vi "Mass Compile Helper.vi"() -> ()   [LabVIEW 2011, in "LVH-Toolbox.lvlib" / "LVH-SystemTools.lvlib"]
uses:
  LVH-SystemTools.lvlib
panel:
  in  "Error In":errorcluster
  out "Error Out":errorcluster
  # "Mass Compiling...."
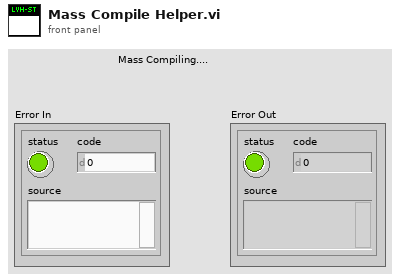
[diagram p1: front panel]
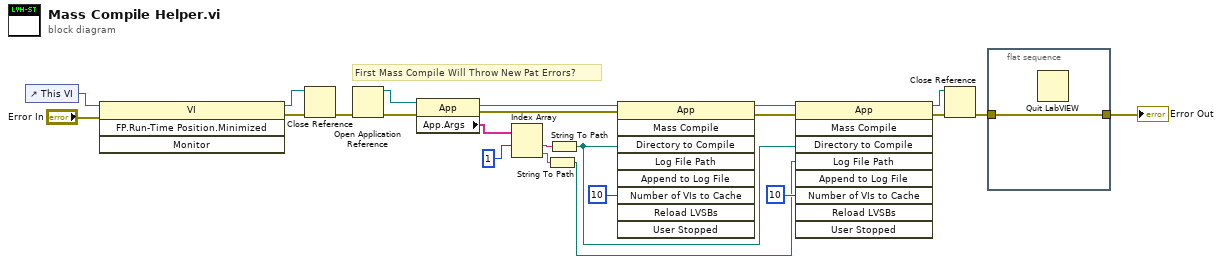
[diagram p0: block diagram]
diagram:
  # "First Mass Compile Will Throw New Pat Errors?"
  n1 = control-ref of="This VI"() -> (w5:refnum<vi>)
  n2 = invoke class="VI" method="FP.Run-Time Position.Minimized"(reference=w5, error in="Error In") -> (reference out=w2:refnum<vi>, error out=w3:errorcluster)  [unwired: 2 in, 2 out]
  n3 = Close Reference(reference=w2, error in (no error)=w3) -> (error out=w1:errorcluster)
  n4 = Open Application Reference(8:w1) -> (0:w13:errorcluster, 3:w15:refnum<vi>)  [unwired: 3 in]
  n5 = property class="App"(reference=w15, error in=w13) -> (reference out=w14:refnum<vi>, error out=w12:errorcluster, "App.Args"=w11:string[])
  n6 = Index Array(array=w11, index #1=1 ("index")) -> (element #1=w7:string, element #2=w6:string)  [unwired: 1 in]
  n7 = String To Path(string=w6) -> (path=w8:path)
  n8 = String To Path(string=w7) -> (path=w9:path)
  n9 = invoke class="App" method="Mass Compile"(reference=w14, error in=w12, "Directory to Compile"=w9, "Number of VIs to Cache"=u32 10) -> (reference out=w22:refnum<vi>, error out=w23:errorcluster)  [unwired: 5 in, 7 out]
  n10 = invoke class="App" method="Mass Compile"(reference=w22, error in=w23, "Directory to Compile"=w9, "Log File Path"=w8, "Number of VIs to Cache"=u32 10) -> (reference out=w20:refnum<vi>, error out=w21:errorcluster)  [unwired: 4 in, 7 out]
  n11 = Close Reference(reference=w20, error in (no error)=w21) -> (error out=w16:errorcluster)
  n12 = flat-sequence {
    tunnel: [w24] -> w17
    tunnel: w16 -> [w24]
    frame #0 {
      n13 = Quit LabVIEW() -> ()  [unwired: 1 in]
    }
  }
  "Error Out" <- w17
